vi "Material-ConfigPage-Initialized.vi"(0 "Configuration Page":refnum<class "Material-ConfigPage.lvclass">, 5 "Allow user to open Diagram from SubPanel?":bool, 11 "error in":errorcluster) -> (4 "Configuration Page out":refnum<class "Material-ConfigPage.lvclass">, 15 "error out":errorcluster)   [LabVIEW 2013, in "Material-ConfigPage.lvclass"]
uses:
  Material-ConfigPage.lvclass
panel:
  # "Inputs"
  # "Outputs"
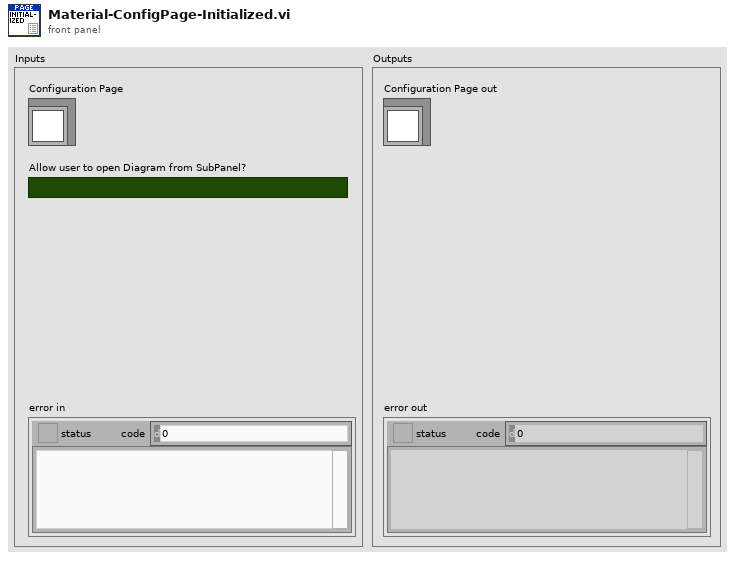
[diagram p1: front panel]
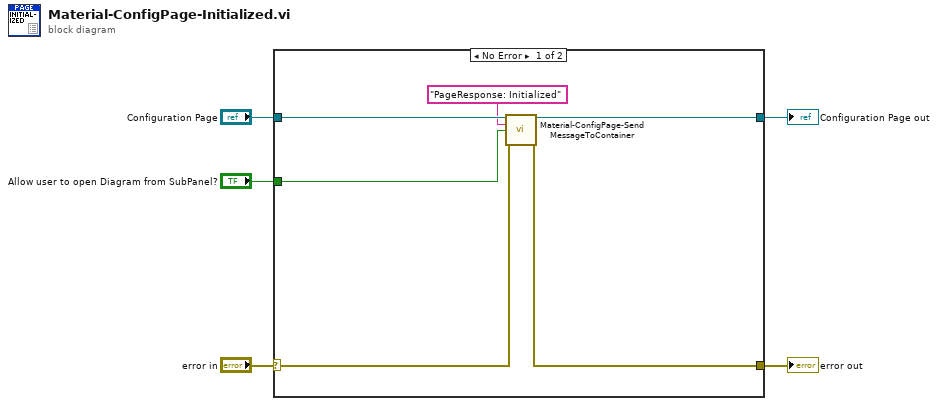
[diagram p0: block diagram]
diagram:
  n1 = case shown="No Error" "error in" {
    selector: "error in" -> [w8 w13]
    tunnel: [w7 w13] -> w5
    tunnel: [w10 w12] -> w3
    tunnel: "Configuration Page" -> [w11 w12]
    tunnel: "Allow user to open Diagram from SubPanel?" -> [w6 _]
    frame No Error {
      n2 = call "Material-ConfigPage-SendMessageToContainer.vi"("Configuration Page"=w11, "Parameter"="PageResponse: Initialized", "Payload"=w6, "error in"=w8) -> ("Configuration Page out"=w10:refnum<class "Material-ConfigPage.lvclass">, "error out"=w7:errorcluster)  [unwired: 10 in]
    }
    frame Error {
    }
  }
  "error out" <- w5
  "Configuration Page out" <- w3
